vi "Esophageal_Datalogger_Initialize.vi"(6 "Python Module Path":path=path "C:/Users/HRME5/Desktop/Multi_Task_Network/compresseddata/mainv6.py", 7 "Data File Path":path, 8 "error in (no error)":errorcluster, 9 "MTN Threshold":dbl, 10 "Patient ID":string, 11 "Log File In":refnum<file>) -> (0 "error out":errorcluster, 3 "Log File Out":refnum<file>)   [LabVIEW 2021]
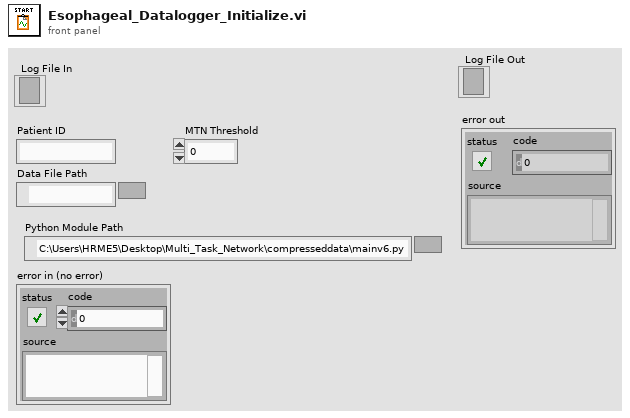
[diagram p1: front panel]
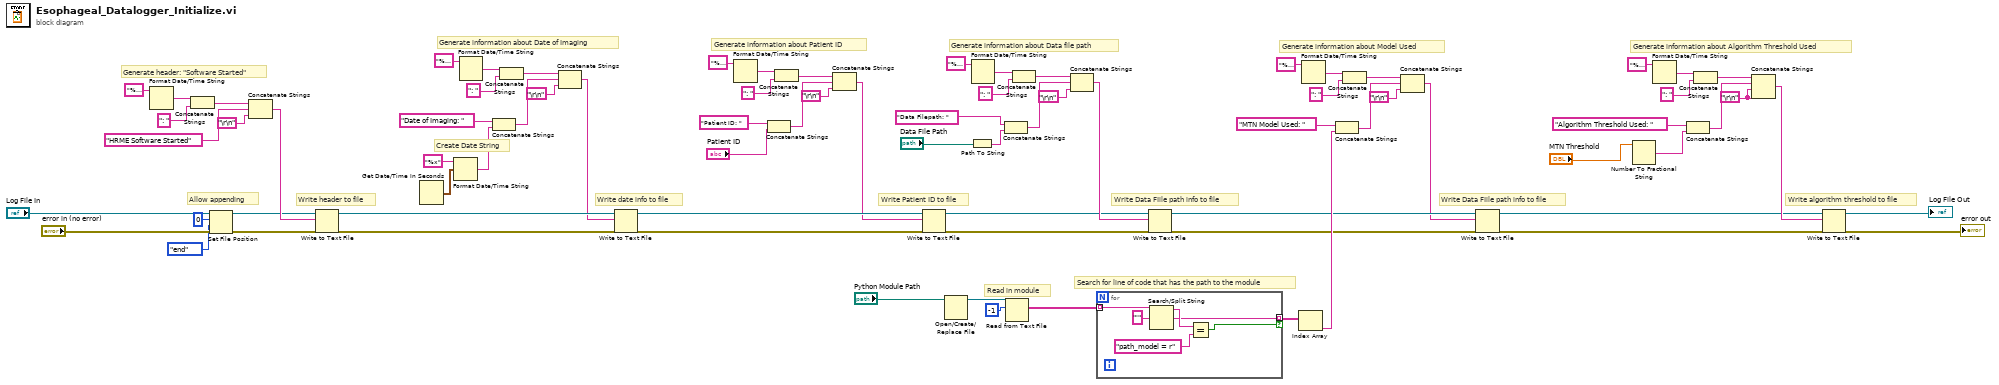
[diagram p0: block diagram]
diagram:
  w3 = "\r\n"
  # "Search for line of code that has the path to the module"
  # "Read in module"
  # "Write Data FIile path info to file"
  # "Generate information about Algorithm Threshold Used"
  # "Write algorithm threshold to file"
  # "Write Data FIile path info to file"
  # "Create Date String"
  # "Generate information about Model Used"
  # "Generate information about Date of Imaging"
  # "Generate information about Data file path"
  # "Generate information about Patient ID"
  # "Write date info to file"
  # "Write header to file"
  # "Generate header: \"Software Started\""
  # "Write Patient ID to file"
  # "Allow appending"
  n1 = Format Date/Time String(time format string (%c)="%H%M%S%3u") -> (date/time string=w64:string)  [unwired: 2 in]
  n2 = Concatenate Strings(w64, ": " ("string")) -> (w66:string)
  n3 = Set File Position(offset (in bytes) (0)=i64 0, refnum="Log File In", from (0:start)=enum16{"start", "end", "current"}."end", error in="error in (no error)") -> (refnum out=w62:refnum<file>, error out=w70:errorcluster)
  n4 = Concatenate Strings(w66, "HRME Software Started" ("time format string (%c)"), "\r\n") -> (w69:string)
  n5 = Write to Text File(file (use dialog)=w62, text=w69, error in=w70) -> (refnum out=w76:refnum<file>, error out=w77:errorcluster)  [unwired: 1 in, 1 out]
  n6 = Get Date/Time In Seconds() -> (seconds since 1Jan1904=w32:timestamp)
  n7 = Format Date/Time String(time format string (%c)="%x", seconds (now)=w32) -> (date/time string=w31:string)  [unwired: 1 in]
  n8 = Format Date/Time String(time format string (%c)="%H%M%S%3u") -> (date/time string=w43:string)  [unwired: 2 in]
  n9 = Concatenate Strings("Date of Imaging: " ("time format string (%c)"), w31) -> (w48:string)
  n10 = Concatenate Strings(w43, ": " ("string")) -> (w45:string)
  n11 = Concatenate Strings(w45, w48, "\r\n") -> (w34:string)
  n12 = Write to Text File(file (use dialog)=w76, text=w34, error in=w77) -> (refnum out=w78:refnum<file>, error out=w79:errorcluster)  [unwired: 1 in, 1 out]
  n13 = Format Date/Time String(time format string (%c)="%H%M%S%3u") -> (date/time string=w74:string)  [unwired: 2 in]
  n14 = Concatenate Strings("Patient ID: " ("time format string (%c)"), "Patient ID") -> (w56:string)
  n15 = Concatenate Strings(w74, ": " ("string")) -> (w72:string)
  n16 = Concatenate Strings(w72, w56, "\r\n") -> (w30:string)
  n17 = Write to Text File(file (use dialog)=w78, text=w30, error in=w79) -> (refnum out=w25:refnum<file>, error out=w24:errorcluster)  [unwired: 1 in, 1 out]
  n18 = Open/Create/Replace File(file path (use dialog)="Python Module Path") -> (refnum out=w11:refnum<file>)  [unwired: 5 in, 2 out]
  n19 = Path To String(path="Data File Path") -> (string=w29:string)
  n20 = Format Date/Time String(time format string (%c)="%H%M%S%3u") -> (date/time string=w50:string)  [unwired: 2 in]
  n21 = Concatenate Strings("Data Filepath: " ("time format string (%c)"), w29) -> (w54:string)
  n22 = Read from Text File(file (use dialog)=w11, count=-1) -> (text=w9:string[])  [unwired: 2 in, 3 out]
  n23 = Concatenate Strings(w50, ": " ("string")) -> (w52:string)
  n24 = Concatenate Strings(w52, w54, "\r\n") -> (w26:string)
  n25 = for {
    tunnel: w9 -> [w85] mode=indexing
    tunnel: [w81] -> w8 mode=indexing if=w80
    n26 = Search/Split String(string=w85, search string/char (-)="'") -> (substring before match=w83:string, match + rest of string=w81:string)  [unwired: 1 in, 1 out]
    n27 = Equal?(x=w83, y="path_model = r") -> (x = y?=w80:bool)
  }
  n28 = Write to Text File(file (use dialog)=w25, text=w26, error in=w24) -> (refnum out=w6:refnum<file>, error out=w5:errorcluster)  [unwired: 1 in, 1 out]
  n29 = Index Array(array=w8) -> (element=w7:string)  [unwired: 1 in]
  n30 = Format Date/Time String(time format string (%c)="%H%M%S%3u") -> (date/time string=w40:string)  [unwired: 2 in]
  n31 = Concatenate Strings("MTN Model Used: " ("time format string (%c)"), w7) -> (w35:string)
  n32 = Concatenate Strings(w40, ": " ("string")) -> (w38:string)
  n33 = Concatenate Strings(w38, w35, "\r\n") -> (w4:string)
  n34 = Write to Text File(file (use dialog)=w6, text=w4, error in=w5) -> (refnum out=w2:refnum<file>, error out=w1:errorcluster)  [unwired: 1 in, 1 out]
  n35 = Number To Fractional String(number="MTN Threshold") -> (F-format string=w15:string)  [unwired: 3 in]
  n36 = Format Date/Time String(time format string (%c)="%H%M%S%3u") -> (date/time string=w17:string)  [unwired: 2 in]
  n37 = Concatenate Strings("Algorithm Threshold Used: " ("time format string (%c)"), w15) -> (w21:string)
  n38 = Concatenate Strings(w17, ": " ("string")) -> (w19:string)
  n39 = Concatenate Strings(w19, w21, w3, w3) -> (w13:string)
  n40 = Write to Text File(file (use dialog)=w2, text=w13, error in=w1) -> (refnum out=→"Log File Out":refnum<file>, error out=→"error out":errorcluster)  [unwired: 1 in, 1 out]
